vi "Destroy.vi"(8 "error in (no error)":errorcluster, 11 "Mock Sift Proxy Server in":refnum<class "Mock Sift Proxy Server.lvclass">) -> (0 "error out":errorcluster, 3 "Mock Sift Proxy Server out":refnum<class "Mock Sift Proxy Server.lvclass">)   [LabVIEW 2024, in "Mock Sift Proxy Server.lvclass"]
uses:
  Mock Sift Proxy Server.lvclass
  Mock Sift Proxy Server.lvclass/Mock Sift Proxy Server.ctl
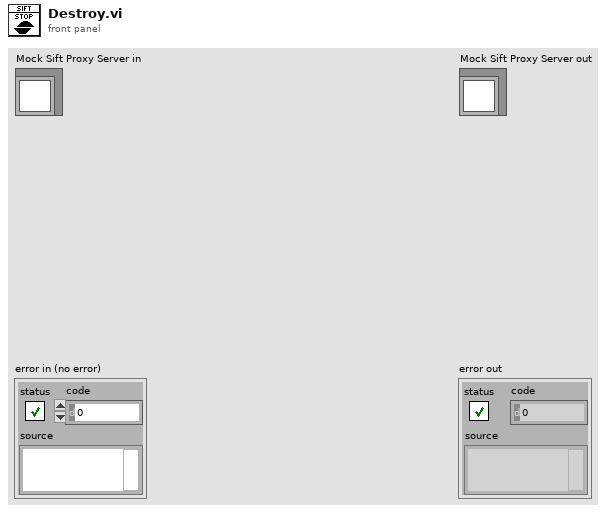
[diagram p1: front panel]
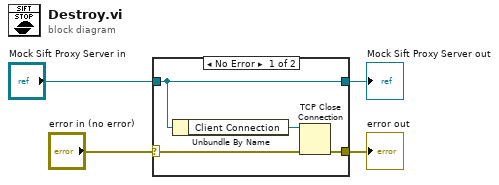
[diagram p0: block diagram]
diagram:
  n1 = case shown="No Error" "error in (no error)" {
    selector: "error in (no error)" -> [w6 w10]
    tunnel: [w5 w10] -> w3
    tunnel: [w8 w9] -> w1
    tunnel: "Mock Sift Proxy Server in" -> [w8 w9]
    frame No Error {
      n2 = Unbundle By Name(w8) -> ("Client Connection"=w7:refnum<k5>)
      n3 = TCP Close Connection(connection ID=w7, error in (no error)=w6) -> (error out=w5:errorcluster)  [unwired: 1 in, 1 out]
    }
    frame Error {
    }
  }
  "error out" <- w3
  "Mock Sift Proxy Server out" <- w1
